vi "signalProcessing.vi"() -> ()   [LabVIEW 2014]
uses:
  <vilib>/express/express analysis/Spectral/Block/exnSpectralBlock spectral measurements RMS poly.vi
  <vilib>/express/express analysis/Spectral/Block/exnSpectralBlock spectral measurements RMS DDT.vi
  <vilib>/express/express analysis/Spectral/XNode/ExpressSpectralMeasurementsBlockNode.xnode
panel:
  out "Error Indicator":errorcluster
  in  "Stop Running":bool
  in  "Frequency 2":dbl(knob) scale=0.0..500.0
  in  "Frequency 1":dbl(knob) scale=0.0..500.0
  in  "Amplitude 2":dbl(knob) scale=0.0..10.0
  in  "Amplitude 1":dbl(knob) scale=0.0..10.0
  out "TimeDomain":dynamicdata(graph)
  out "Frequency Domain":dynamicdata(graph)
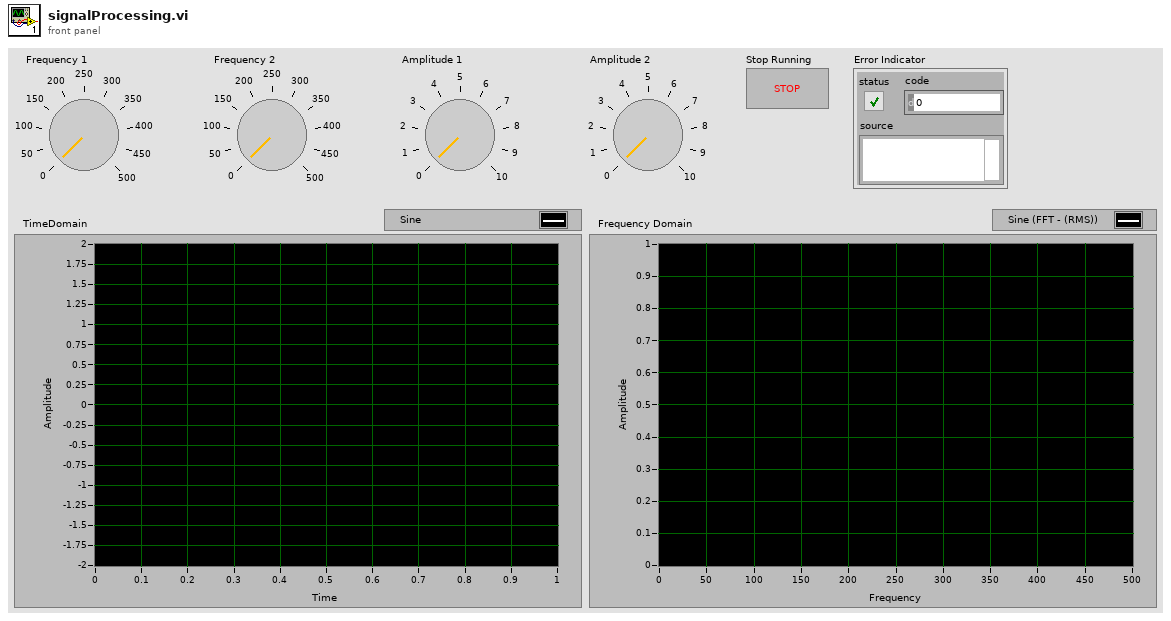
[diagram p1: front panel]
types:
  T1 = cluster{"averaging mode":u16, "weighting mode":u16, "number of averages":u32}
  T2 = cluster{"dB On (F)":bool, "unwrap phase (F)":bool, "convert to degree (F)":bool}
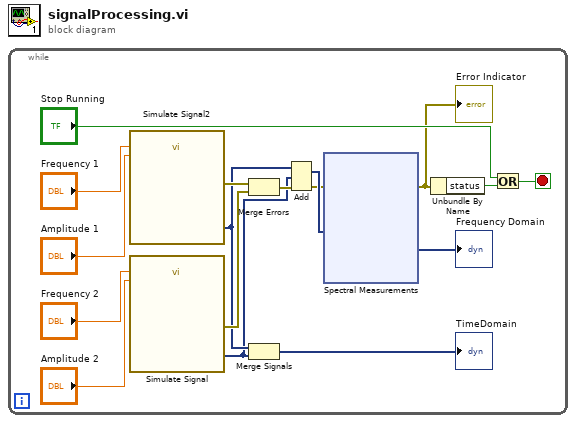
[diagram p0: block diagram]
diagram:
  n1 = while {
    stop <- w3 stop-if-true
    n2 = call "Simulate Signal2"("Frequency"="Frequency 1", "Amplitude"="Amplitude 1") -> ("Sine"=w7:dynamicdata, "error out"=w11:errorcluster)  [unwired: 12 in]
    n3 = call "Simulate Signal"("Frequency"="Frequency 2", "Amplitude"="Amplitude 2") -> ("Sine with Uniform Noise"=w6:dynamicdata, "error out"=w10:errorcluster)  [unwired: 12 in]
    n4 = Merge Errors(w11, w10) -> (w9:errorcluster)
    n5 = Merge Signals(w7, w6) -> (→"TimeDomain":dynamicdata)
    n6 = Add(1:w6, 2:w7, 4:w9) -> (0:w16:dynamicdata, 3:w8:errorcluster)
    n7 = xnode "Spectral Measurements"("Signals"=w16, "error in (no error)"=w8) -> ("FFT - (RMS)"=→"Frequency Domain":dynamicdata, "error out"=w2:errorcluster)  [unwired: 1 out]
    "Error Indicator" <- w2
    n8 = Unbundle By Name(w2) -> ("status"=w1:bool)
    n9 = Or(x="Stop Running", y=w1) -> (x .or. y?=w3:bool)
  }
